vi "DebugActions.vi"(5 "KeepOpen":bool, 6 "DebugOn":bool, 7 "ThisVI":refnum<vi>, 8 "ErrorIn":errorcluster, 9 "CmdData":variant, 10 "VIIn":refnum<vi>, 11 "Continue":refnum<vi>) -> (0 "ErrorOut":errorcluster, 2 "XmlString":string)   [LabVIEW 2021, in "YActor.lvclass"]
uses:
  YActor.lvclass
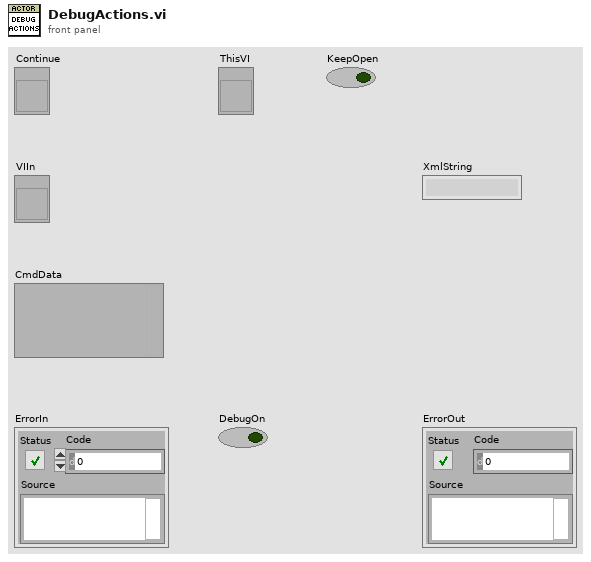
[diagram p1: front panel]
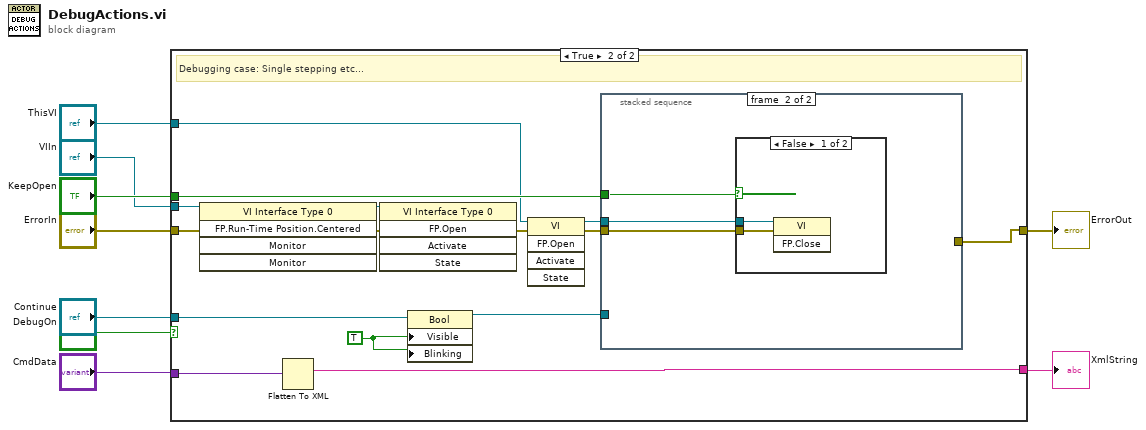
[diagram p0: block diagram]
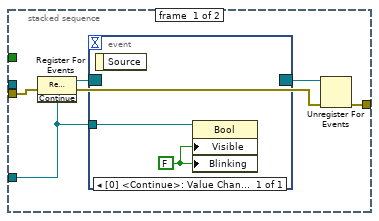
[diagram p3: hidden frame]
diagram:
  n1 = case shown="True" "DebugOn" {
    tunnel: "VIIn" -> [_ w19]
    tunnel: "ErrorIn" -> [w10 w23]
    tunnel: [w10 w21] -> w9
    tunnel: "CmdData" -> [_ w20]
    tunnel: "Continue" -> [_ w16]
    tunnel: "ThisVI" -> [_ w13]
    tunnel: "KeepOpen" -> [_ w14]
    tunnel: [_ w12] -> w7
    frame False {
      # "Normal operation"
    }
    frame True {
      w17 = TRUE ("Visible")
      # "Debugging case: Single stepping etc..."
      n2 = invoke class="VI Interface Type 0" method="FP.Run-Time Position.Centered"(reference=w19) -> (reference out=w18:refnum<vi>)  [unwired: 4 in, 4 out]
      n3 = Flatten To XML(6:w20) -> (2:w12:string)
      n4 = invoke class="VI Interface Type 0" method="FP.Open"(reference=w18) -> ()  [unwired: 4 in, 5 out]
      n5 = property on="Property Node" class="Bool"(reference=w16, "Visible"=w17, "Blinking"=w17) -> (reference out=w15:refnum<vi>)  [unwired: 1 in, 1 out]
      n6 = invoke class="VI" method="FP.Open"(reference=w13, error in=w23) -> (reference out=w11:refnum<vi>, error out=w22:errorcluster)  [unwired: 3 in, 3 out]
      n7 = stacked-sequence {
        tunnel: w15 -> [w26 _]
        tunnel: w14 -> [_ w33]
        tunnel: w11 -> [_ w32]
        tunnel: w22 -> [w29 w34]
        tunnel: [w27 _] -> w21
        frame #0 {
          n8 = register-events(error in=w29, w26) -> (reference out=w25:refnum<event-registration>, error out=w28:errorcluster)  [unwired: 1 in]
          n9 = event shown="[0] <Continue>: Value Change" {
            selector: w25 -> [_]
            dyn-events: [_] -> w24
            timeout: _ -> [_]
            tunnel: w26 -> [w30]
            event Value Change {
              w31 = FALSE ("Visible")
              n10 = event-data() -> ()  [unwired: 1 in, 1 out]
              n11 = property on="Property Node" class="Bool"(reference=w30, "Visible"=w31, "Blinking"=w31) -> ()  [unwired: 1 in, 2 out]
            }
          }
          n12 = Unregister For Events(event registration refnum=w24, error in=w28) -> (error out=w27:errorcluster)
        }
        frame #1 {
          n13 = case shown="False" w33 {
            tunnel: w32 -> [w35 _]
            tunnel: w34 -> [w36 _]
            frame False {
              n14 = invoke class="VI" method="FP.Close"(reference=w35, error in=w36) -> ()  [unwired: 1 in, 3 out]
            }
            frame True {
            }
          }
        }
      }
    }
  }
  "XmlString" <- w7
  "ErrorOut" <- w9
